vi "CoordSystem_NWU.vi"() -> (0 "Error":bool, 3 "out Coordinate System":T1={"Rotation"={"Q_quaternion"={"R"=1.0, "V"=[0.0, 0.0, 0.0]}}})   [LabVIEW 2019, in "Trajectory_Library.lvlib"]
doc: "Convenience constructors that takes in x and y values directly instead of having to construct a Translation2d.\n\nParameters:\n - X- The x component of the translational component of the pose.\n - Y - The y component of the translational component of the pose.\n - Rotation (Heading) - The rotational component of the pose.\n\nReturns:\n - OUT POSE - Output POSE"
uses:
  Trajectory_Library.lvlib
  COORDINATE_SYSTEM.ctl
  ROTATION3D.ctl
  QUATERNION.ctl
  CoordAxis_New.vi
  MatBuilder_Create.vi
  Matrix_AssignBlock.vi
  Matrix_Transpose.vi
  Matrix_Ident.vi
  Matrix_IsEqual.vi
  <vilib>/Analysis/baseanly.llb/A x B.vi
  <vilib>/Analysis/baseanly.llb/Real A x B.vi
  Quaternion_New.vi
  Rotation3d_Create_Quaternion.vi
  MatrixHelper_CoerceSize.vi
  Quaternion_Normalize.vi
  Quaternion_New_Default.vi
  <vilib>/Analysis/7linalg.llb/Create Special Matrix.vi
  <vilib>/Analysis/7linalg.llb/Create Special Real Matrix.vi
  <vilib>/Analysis/Matrix/Numeric/Conversions/Array To Matrix.vi
  <vilib>/Analysis/Matrix/Numeric/Conversions/Array To Matrix - RA.vi
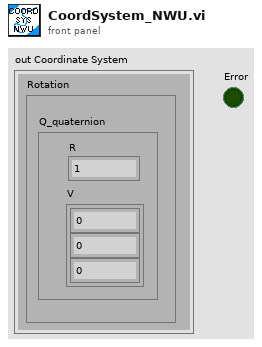
[diagram p1: front panel]
types:
  T1 = typedef "Trajectory_Library.lvlib/COORDINATE_SYSTEM.ctl" = cluster{"Rotation":T2}
  T2 = typedef "Trajectory_Library.lvlib/ROTATION3D.ctl" = cluster{"Q_quaternion":T3}
  T3 = typedef "Trajectory_Library.lvlib/QUATERNION.ctl" = cluster{"R":dbl, "V":dbl[]}
  T4 = typedef "Trajectory_Library.lvlib/COORDINATE_AXIS.ctl" = cluster{"Axis":dbl[]}
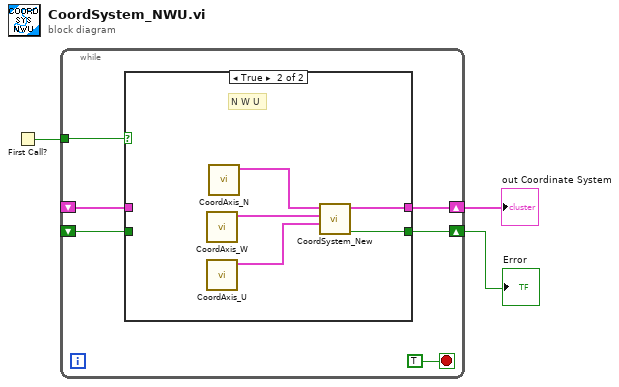
[diagram p0: block diagram]
diagram:
  n1 = First Call?() -> (First Call?: T/F=w1:bool)
  n2 = while {
    shift-right: [w8] -> w2
    shift-left: _ -> [w5]
    shift-right: [w9] -> w3
    shift-left: _ -> [w6]
    tunnel: w1 -> [w7]
    stop <- TRUE stop-if-true
    n3 = case shown="True" w7 {
      tunnel: [w11 w16] -> w9
      tunnel: [w10 w15] -> w8
      tunnel: w6 -> [w11 _]
      tunnel: w5 -> [w10 _]
      frame False {
      }
      frame True {
        # "N W U"
        n4 = call "CoordAxis_W.vi"() -> ("out Coordinate Axis"=w13:T4)  [unwired: 11 in]
        n5 = call "CoordAxis_U.vi"() -> ("out Coordinate Axis"=w12:T4)  [unwired: 11 in]
        n6 = call "CoordAxis_N.vi"() -> ("out Coordinate Axis"=w14:T4)  [unwired: 11 in]
        n7 = call "CoordSystem_New.vi"("PositiveZ"=w12, "PositveY"=w13, "PositiveX"=w14) -> ("Error"=w15:bool, "out Coordinate System"=w16:T1)  [unwired: 7 in]
      }
    }
  }
  "out Coordinate System" <- w3
  "Error" <- w2
